vi "Path_String_Splitter_New.vi"(0 "File Path":path) -> (1 "Experiment Name":string, 2 "Session Name":string, 3 "Experment Index":i32, 4 "Session Index":i32)   [LabVIEW 2023]
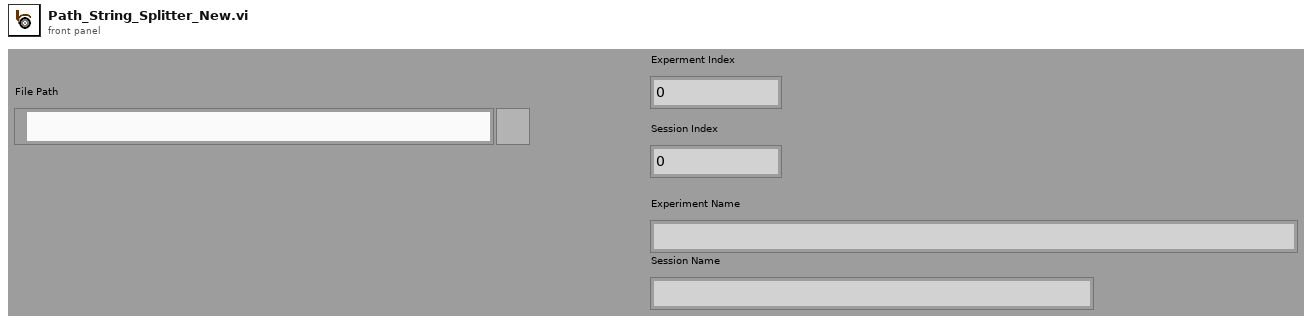
[diagram p1: front panel]
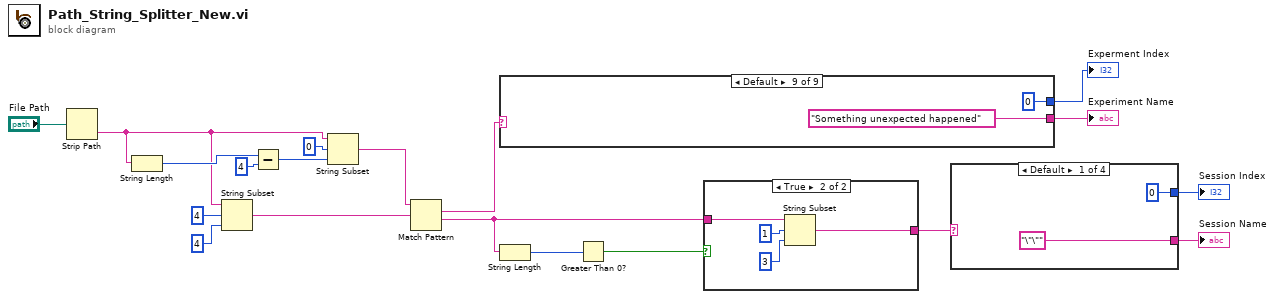
[diagram p0: block diagram]
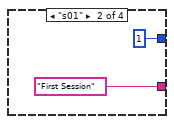
[diagram p2: hidden frame]
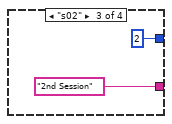
[diagram p3: hidden frame]
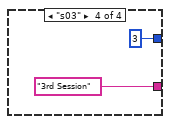
[diagram p4: hidden frame]
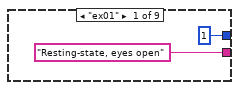
[diagram p5: hidden frame]
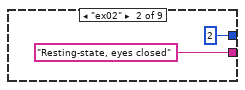
[diagram p6: hidden frame]
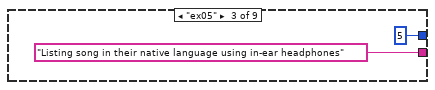
[diagram p7: hidden frame]
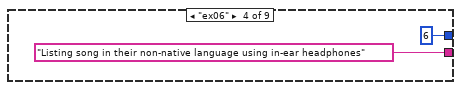
[diagram p8: hidden frame]
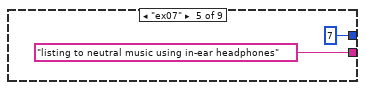
[diagram p9: hidden frame]
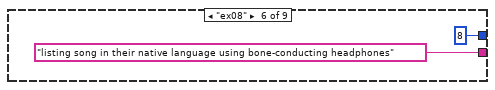
[diagram p10: hidden frame]
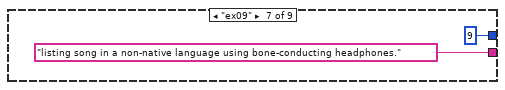
[diagram p11: hidden frame]
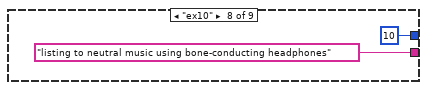
[diagram p12: hidden frame]
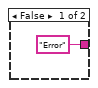
[diagram p13: hidden frame]
diagram:
  n1 = Strip Path(path="File Path") -> (name=w10:string)  [unwired: 1 out]
  n2 = String Length(string=w10) -> (length=w17:i32)
  n3 = String Subset(string=w10, offset (0)=4, length (rest)=4 ("length (rest)")) -> (substring=w7:string)
  n4 = Subtract(x=w17, y=4) -> (x-y=w19:i32)
  n5 = String Subset(string=w10, offset (0)=0, length (rest)=w19) -> (substring=w16:string)
  n6 = Match Pattern(string=w16, regular expression=w7) -> (match substring=w6:string, after substring=w13:string)  [unwired: 1 in, 2 out]
  n7 = case shown="Default" w6 {
    tunnel: [1 2 5 6 7 8 9 10 0] -> w4
    tunnel: ["Resting-state, eyes open" "Resting-state, eyes closed" "Listing song in their native language using in-ear headphones" "Listing song in their non-native language using in-ear headphones" "listing to neutral music using in-ear headphones" "listing song in their native language using bone-conducting headphones" "listing song in a non-native language using bone-conducting headphones." "listing to neutral music using bone-conducting headphones" "Something unexpected happened"] -> w2
    frame "ex01" {
    }
    frame "ex02" {
    }
    frame "ex05" {
    }
    frame "ex06" {
    }
    frame "ex07" {
    }
    frame "ex08" {
    }
    frame "ex09" {
    }
    frame "ex10" {
    }
    frame Default {
    }
  }
  "Experment Index" <- w4
  "Experiment Name" <- w2
  n8 = String Length(string=w13) -> (length=w12:i32)
  n9 = Greater Than 0?(x=w12) -> (x > 0?=w11:bool)
  n10 = case shown="True" w11 {
    tunnel: w13 -> [_ w40]
    tunnel: ["Error" w39] -> w5
    frame False {
    }
    frame True {
      n11 = String Subset(string=w40, offset (0)=1, length (rest)=3 ("length (rest)")) -> (substring=w39:string)
    }
  }
  n12 = case shown="Default" w5 {
    tunnel: [0 1 2 3] -> w3
    tunnel: ["\"\"" "First Session" "2nd Session" "3rd Session"] -> w1
    frame Default {
    }
    frame "s01" {
    }
    frame "s02" {
    }
    frame "s03" {
    }
  }
  "Session Index" <- w3
  "Session Name" <- w1
